vi "DHE_Modifiers2Str.vi"() -> (2 "modifiers":string)   [LabVIEW 2016]
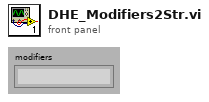
[diagram p1: front panel]
types:
  T1 = typedef "GEOM_AmpModifiers.ctl" = cluster{"Binning":T2, "sections":T3[]}
  T2 = typedef "GEOM_Binning.ctl" = cluster{"x":u32, "y":u32}
  T3 = typedef "GEOM_Moifier.ctl" = cluster{"name":string, "header section":string, "comment":string, "value":i32, "binning?":bool, "Where":enum16{"predata", "postdata"}, "add In":enum16{"columns", "rows", "none"}}
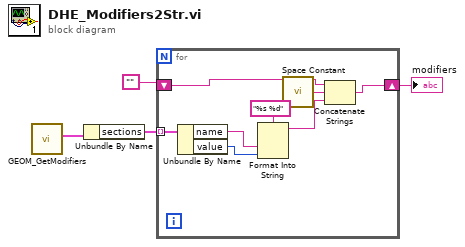
[diagram p0: block diagram]
diagram:
  n1 = call "GEOM_GetModifiers.vi"() -> ("GEOM_modifiers"=w4:T1)  [unwired: 1 in, 10 out]
  n2 = Unbundle By Name(w4) -> ("sections"=w3:T3[])
  n3 = for {
    tunnel: w3 -> [w12] mode=indexing
    shift-right: [w6] -> w1
    shift-left: "" -> [w5]
    n4 = Unbundle By Name(w12) -> ("name"=w11:string, "value"=w10:i32)
    n5 = Format Into String(format string="%s %d", w11, w10) -> (resulting string=w8:string)  [unwired: 2 in, 1 out]
    n6 = call <vilib>:"Space Constant.vi"() -> ("String"=w7:string)
    n7 = Concatenate Strings(w5, w7, w8) -> (w6:string)
  }
  "modifiers" <- w1
